vi "nValue.vi"(6 "Numeric 3":dbl, 9 "nCarrot":dbl, 10 "Numeric 2":dbl, 11 "Numeric":dbl) -> (3 "n":dbl)   [LabVIEW 2020]
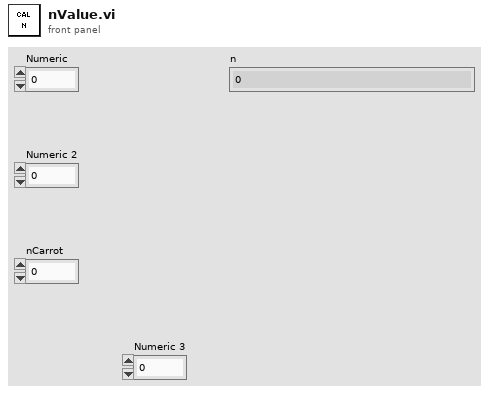
[diagram p1: front panel]
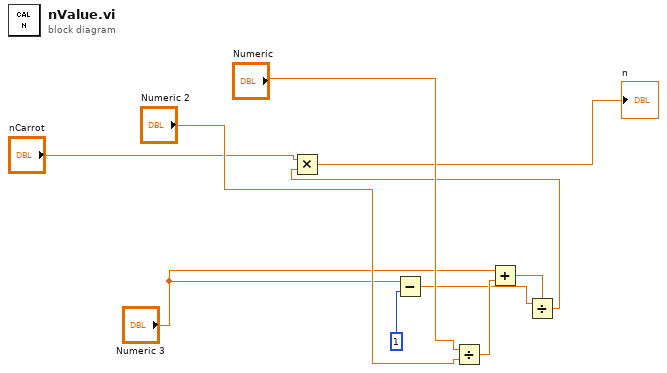
[diagram p0: block diagram]
diagram:
  n1 = Subtract(x="Numeric 3", y=1) -> (x-y=w2:dbl)
  n2 = Divide(x="Numeric", y="Numeric 2") -> (x/y=w4:dbl)
  n3 = Add(x="Numeric 3", y=w4) -> (x+y=w5:dbl)
  n4 = Divide(x=w2, y=w5) -> (x/y=w6:dbl)
  n5 = Multiply(x="nCarrot", y=w6) -> (x*y=→"n":dbl)
